vi "GetReceiveNum.vi"(8 "error in (no error)":errorcluster caption="错误输入（无错误）", 9 "CANInd":u32, 10 "DeciceInd":u32, 11 "DeviceType":u32) -> (0 "error out":errorcluster caption="错误输出", 3 "FrmsUnRead":u32)   [LabVIEW 2011]
uses:
  data/ControlCAN.dll
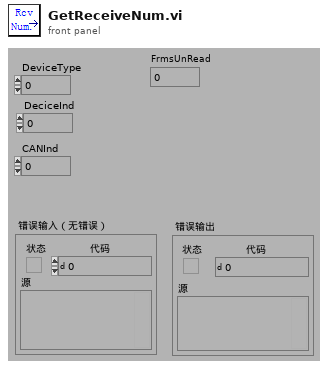
[diagram p1: front panel]
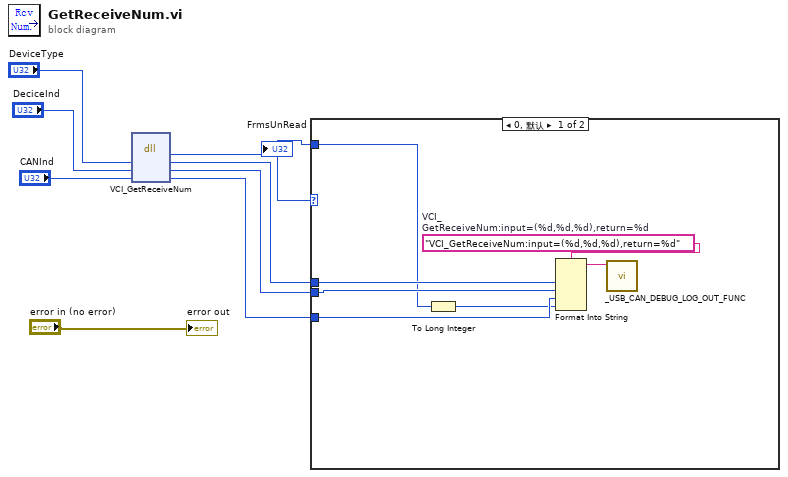
[diagram p0: block diagram]
diagram:
  n1 = dll-call lib="PTH1Mabs ZHost_E工作TnewcodeUSB CAN Tool1.97dataControlCAN.dll" fn="VCI_GetReceiveNum"("DeviceType"="DeviceType", "DeciceInd"="DeciceInd", "CANInd"="CANInd") -> ("返回类型"=w1:u32, "DeviceType"=w4:u32, "DeciceInd"=w3:u32, "CANInd"=w2:u32)  [unwired: 3 in, 2 out]
  "FrmsUnRead" <- w1
  n2 = case shown="0, 默认" w1 {
    tunnel: w4 -> [w14 _]
    tunnel: w3 -> [w13 _]
    tunnel: w1 -> [w12 _]
    tunnel: w2 -> [w11 _]
    frame 0, Default {
      w9 = "VCI_GetReceiveNum:input=(%d,%d,%d),return=%d"  # VCI_GetReceiveNum:input=(%d,%d,%d),return=%d
      n3 = To Long Integer(number=w12) -> (32bit integer=w10:i32)
      n4 = Format Into String(format string=w9, w14, w13, w11, w10) -> (resulting string=w15:string)  [unwired: 2 in, 1 out]
      n5 = call "_USB_CAN_DEBUG_LOG_OUT_FUNC.vi"("Info"=w15) -> ()  [unwired: 11 in]
    }
    frame 1 {
    }
  }
  "error out" <- "error in (no error)"
